vi "Get Error.vi"(8 "error in":errorcluster, 11 "LogRecord in":refnum<class "LogRecord.lvclass">) -> (0 "error out":errorcluster, 2 "Error":errorcluster, 3 "LogRecord out":refnum<class "LogRecord.lvclass">)   [LabVIEW 2020, in "hse-logger.lvlib" / "LogRecord.lvclass"]
doc: "Returns the error-cluster from the LogRecord.\n\n____\nHAMPEL SOFTWARE ENGINEERING v2.0.6 (2021-04-15 11:38)"
uses:
  LogRecord.lvclass
  LogRecord.lvclass/LogRecord.ctl
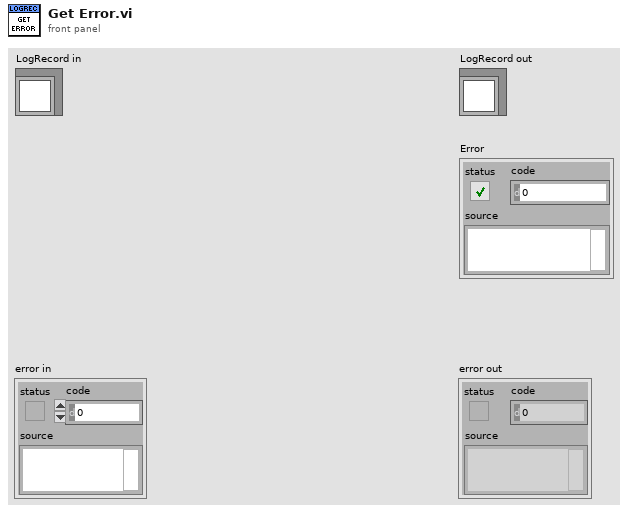
[diagram p1: front panel]
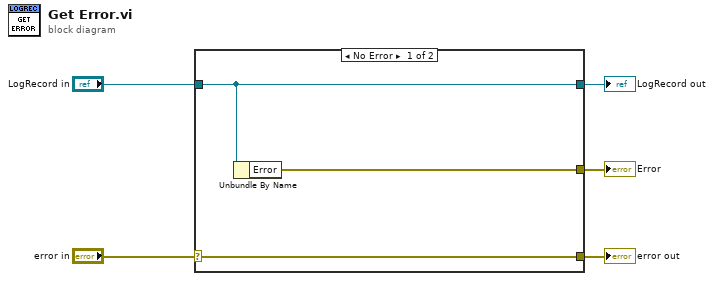
[diagram p0: block diagram]
diagram:
  n1 = case shown="No Error" "error in" {
    selector: "error in" -> [w8 w9]
    tunnel: [w8 w9] -> w4
    tunnel: [w7 w10] -> w2
    tunnel: "LogRecord in" -> [w7 w10]
    tunnel: [w6 _] -> w1
    frame No Error {
      n2 = Unbundle By Name(w7) -> ("Error"=w6:errorcluster)
    }
    frame Error {
    }
  }
  "error out" <- w4
  "LogRecord out" <- w2
  "Error" <- w1
